vi "ATF Storage-Seq Execution Monitor.vi"(8 "error in":errorcluster, 9 "Seq Monitor":string[](array[string]), 11 "Enum":enum16{"Read", "Write "}(ring)) -> (0 "error out":errorcluster, 1 "Seq Monitor":string[](array[string]))   [LabVIEW 2022 SP3]
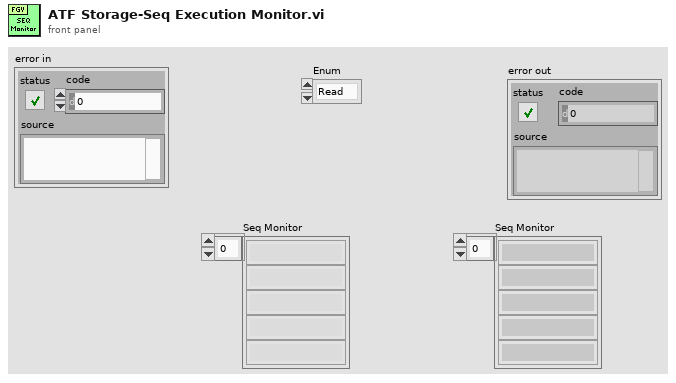
[diagram p1: front panel]
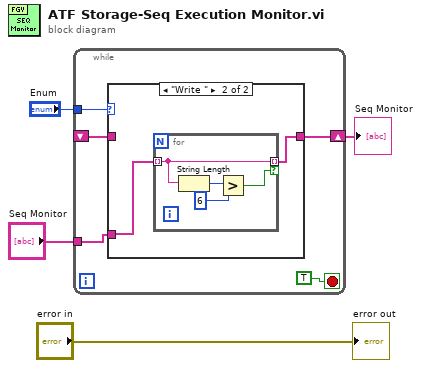
[diagram p0: block diagram]
diagram:
  n1 = while {
    tunnel: "Enum" -> [w9]
    tunnel: "Seq Monitor" -> [w7]
    shift-right: [w6] -> w1
    shift-left: _ -> [w5]
    stop <- TRUE stop-if-true
    n2 = case shown="\"Write \"" w9 {
      tunnel: w7 -> [_ w12]
      tunnel: [w10 w11] -> w6
      tunnel: w5 -> [w10 _]
      frame "Read", Default {
      }
      frame "Write " {
        n3 = for {
          tunnel: w12 -> [w14] mode=indexing
          tunnel: [w14] -> w11 mode=indexing if=w13
          n4 = String Length(string=w14) -> (length=w16:i32)
          n5 = Greater?(x=w16, y=6) -> (0:w13:bool)
        }
      }
    }
  }
  "Seq Monitor" <- w1
  "error out" <- "error in"
